vi "DistancePointLine.vi"(7 "Q":dbl[](array[numeric]), 8 "error in (no error)":errorcluster, 9 "P2":dbl[](array[numeric]), 10 "P1":dbl[](array[numeric]), 11 "Utilities in":refnum<class "Utilities.lvclass">) -> (0 "error out":errorcluster, 2 "distance":dbl, 3 "Utilities out":refnum<class "Utilities.lvclass">)   [LabVIEW 2020, in "Utilities.lvclass"]
uses:
  Utilities.lvclass
  <vilib>/Analysis/_algsub.llb/Real Vector Norm.vi
  <vilib>/Analysis/NI_AALPro.lvlib
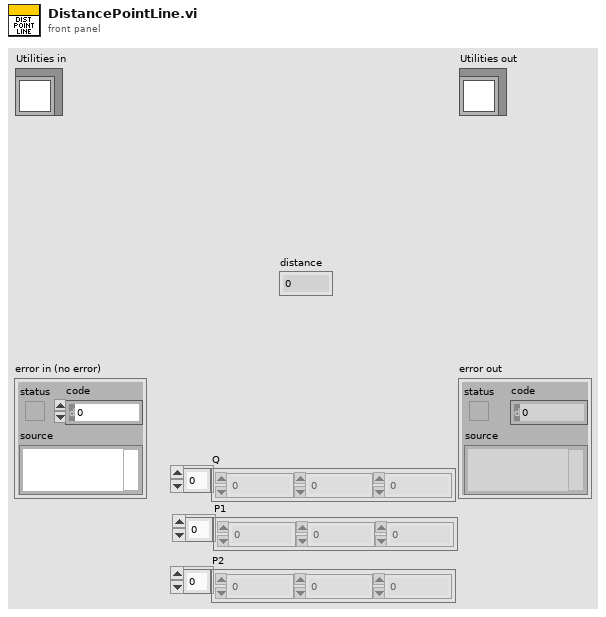
[diagram p1: front panel]
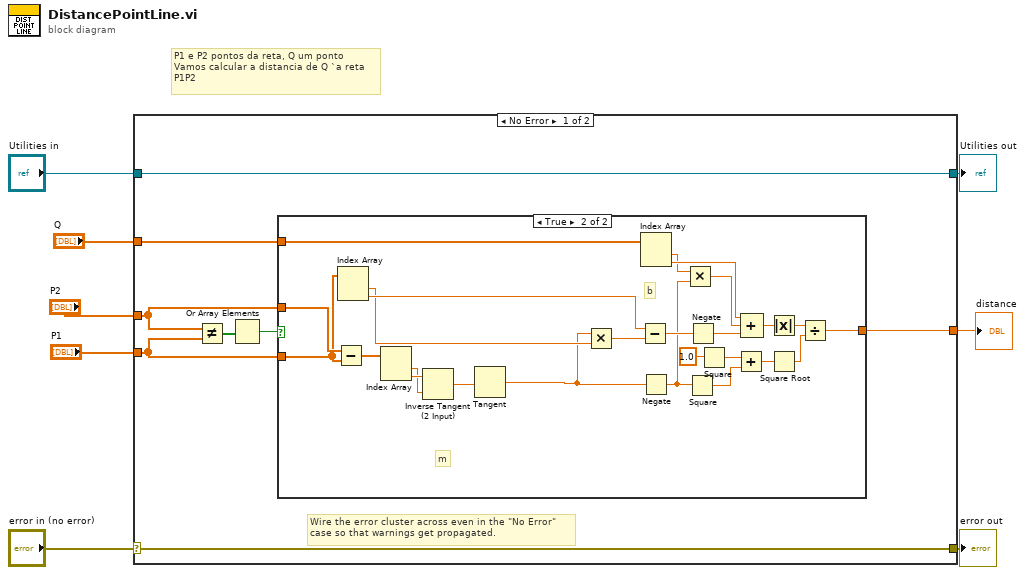
[diagram p0: block diagram]
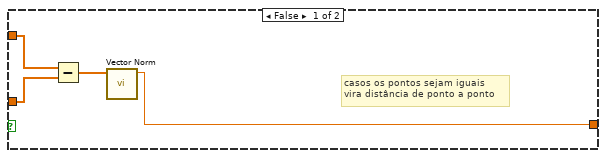
[diagram p2: hidden frame]
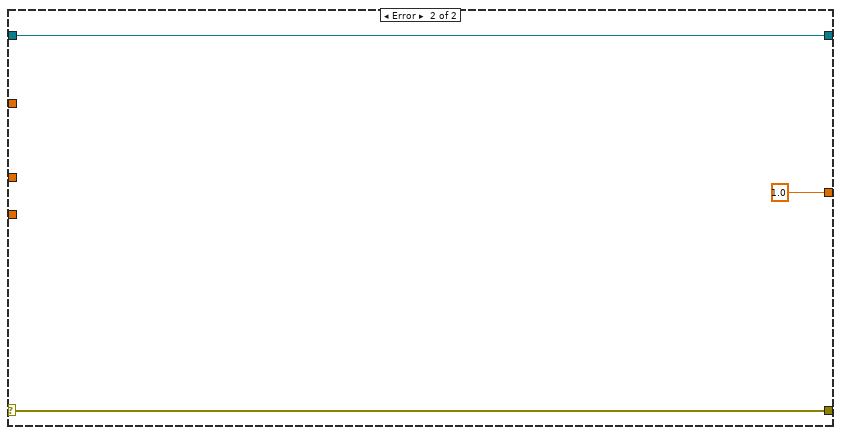
[diagram p3: hidden frame]
diagram:
  # "P1 e P2 pontos da reta, Q um ponto\nVamos calcular a distancia de Q `a reta \nP1P2"
  n1 = case shown="No Error" "error in (no error)" {
    selector: "error in (no error)" -> [w15 w48]
    tunnel: [w15 w48] -> w7
    tunnel: [w16 w47] -> w5
    tunnel: "Utilities in" -> [w16 w47]
    tunnel: [w12 1.0] -> w4
    tunnel: "Q" -> [w11 _]
    tunnel: "P2" -> [w10 _]
    tunnel: "P1" -> [w9 _]
    frame No Error {
      # "Wire the error cluster across even in the \"No Error\"\ncase so that warnings get propagated."
      n2 = Not Equal?(x=w10, y=w9) -> (x != y?=w14:bool[])
      n3 = Or Array Elements(Boolean array=w14) -> (logical OR=w13:bool)
      n4 = case shown="True" w13 {
        tunnel: w10 -> [w19 w45]
        tunnel: w9 -> [_ w41]
        tunnel: w11 -> [w20 w37]
        tunnel: [w17 w23] -> w12
        frame False {
          # "casos os pontos sejam iguais\nvira distância de ponto a ponto"
          n5 = Subtract(x=w20, y=w19) -> (x-y=w18:dbl[])
          n6 = call-poly <vilib>:"Vector Norm.vi"("Input Vector"=w18) -> ("norm"=w17:dbl)  [unwired: 9 in, 1 out]
        }
        frame True {
          # "b"
          # "m"
          n7 = Subtract(x=w45, y=w41) -> (x-y=w44:dbl[])
          n8 = Index Array(array=w41) -> (element #1=w39:dbl, element #2=w40:dbl)  [unwired: 2 in]
          n9 = Index Array(array=w44) -> (element #1=w42:dbl, element #2=w43:dbl)  [unwired: 2 in]
          n10 = Inverse Tangent (2 Input)(1:w42, 2:w43) -> (0:w22:dbl)
          n11 = Tangent(1:w22) -> (0:w21:dbl)
          n12 = Multiply(x=w21, y=w39) -> (x*y=w38:dbl)
          n13 = Subtract(x=w40, y=w38) -> (x-y=w33:dbl)
          n14 = Index Array(array=w37) -> (element #1=w35:dbl, element #2=w36:dbl)  [unwired: 2 in]
          n15 = Negate(x=w21) -> (-x=w29:dbl)
          n16 = Multiply(x=w35, y=w29) -> (x*y=w34:dbl)
          n17 = Square(x=w29) -> (x^2=w27:dbl)
          n18 = Negate(x=w33) -> (-x=w32:dbl)
          n19 = Square(x=1.0) -> (x^2=w28:dbl)
          n20 = Add(x=w28, y=w27) -> (x+y=w26:dbl)
          n21 = Compound Arithmetic op=ADD(w36, w34, w32) -> (w31:dbl)
          n22 = Absolute Value(x=w31) -> (abs(x)=w25:dbl)
          n23 = Square Root(x=w26) -> (sqrt(x)=w24:dbl)
          n24 = Divide(x=w25, y=w24) -> (x/y=w23:dbl)
        }
      }
    }
    frame Error {
    }
  }
  "error out" <- w7
  "Utilities out" <- w5
  "distance" <- w4
